vi "Soft_Robot Model.vi"() -> ()   [LabVIEW 2015]
uses:
  <vilib>/addons/Control Design/_Model Construction/Model Typedefs.llb/CD State Space Model (MIMO).ctl
  <vilib>/addons/Control Design/_Model Construction/Model Typedefs.llb/CD General Elements.ctl
  <vilib>/Analysis/Matrix/Datatypes/RealMatrix.ctl
  <vilib>/Platform/TimedLoop/XDataNode/timing_clust.ctl
  <vilib>/Platform/TimedLoop/XDataNode/nitl_modes.ctl
  <vilib>/Platform/TimedLoop/XDataNode/wakeup.ctl
  <vilib>/FPGAPlugInAG/myRIO-1900/niLvFpga_Open_myRIO-1900.vi
  <vilib>/rvi/interface/common/dynamic/niFpgaDynamicAddResources.vi
  <vilib>/Utility/error.llb/Error Cluster From Error Code.vi
  <vilib>/rvi/errors/niLvFpgaAdjustHostInterfaceError.vi
  <vilib>/FPGAPlugInAG/Dynamic/niLvFpga_Close_Dynamic.vi
  <vilib>/addons/Control Design/_Model Construction/Model Creation.llb/Model Creation SubVI/cd_Create State Space Model.vi
  <vilib>/addons/Control Design/_Stochastic Systems/Stochastic Systems.llb/CD Construct Noise Model (Numeric).vi
  <vilib>/Analysis/7linalg.llb/Create Special Real Matrix.vi
  <vilib>/addons/Control Design/_State Feedback Control/State Feedback Control.llb/State Feedback Control SubVis/cd_Linear Quadratic Regulator.vi
  <vilib>/Simulation/Estimation/Implementation/NILVSim Discrete Kalman Filter.llb/SIM Disc KF Pred and Corr with Pred Gain with Checking Direct LV.vi
  <vilib>/rvi/interface/nirviOpenFPGA/nirviOpenFPGA.xnode
  FPGA Bitfiles/ACC20115_FPGATarget_CurrentControlle_Dt5vFgOzYtY.lvbitx
  Current Controller.vi
  <vilib>/rvi/interface/nirviReadWriteControl/nirviReadWriteControl.xnode
  <vilib>/rvi/interface/nirviCloseFPGA/nirviCloseFPGA.xnode
  <vilib>/Platform/TimedLoop/XDataNode/XDataNode.xnode
  <vilib>/Simulation/Implementation/XNodeFramework/SimXNode/SimX.xnode
  NiFpgaLv.dll
  <vilib>/rvi/interface/Simulation/niFpgaSimulationCallBeginRW.vi
  <vilib>/addons/Control Design/_Model Construction/NI_LinSys_Model Creation.lvlib
  <vilib>/addons/Control Design/_State Feedback Control/NI_CD_State Feedback Control.lvlib
  <vilib>/addons/Control Design/_Stochastic Systems/NI_CD_Stochastic Systems.lvlib
  <vilib>/Platform/TimedLoop/XDataNode/XDNodeRunTimeDep.lvlib
  <vilib>/Analysis/NI_AALPro.lvlib
  <vilib>/addons/Control Design/_Model Construction/NI_LinSys_Model Typedefs.lvlib
  <vilib>/Analysis/Matrix/NI_Matrix.lvlib
panel:
  in  "LQR Q":T1
  out "error IO":errorcluster
  in  "Tab Control":enum32{"Outputs/Control", "Model Info"}(tab)
  out "DAC Inlet Valve 2":i32(graph)
  out "Fusion Data":dbl(graph)
  out "KF estimate":dbl[](graph)
  in  "SP1:":dbl(slide)=40.87020302841148 min=0.0 max=0.0 scale=0.0..720.0
  in  "Stop":bool
  in  "LQR Weight (LQR R)":dbl(knob)=1.2163765459278015 scale=1.0..10.0
  out "Status?":bool
  in  "Current (mA)":i32
  out "State-Space Model":T2 {"Transport Delay" format="%.2f"; "D" format="%#.2g"; "C" format="%#.2g"; "B" format="%#.2g"; "A" format="%#.2g"; "properties"."Sampling Time" format="%#.6p"; "properties"."Output Delays" format="%.4f"; "properties"."Input Delays" format="%.4f"}
  in  "A":dbl[][](array[numeric])=[[1.1159, -0.2446, -0.2446, -0.2726], [-0.0103, 0.8088, 0.0684, 0.1117], [-0.167, 0.1085, 0.5344, 0.1174], [0.1346, 0.1551, -0.1383, 0.5146]] format="%#.5g"
  in  "B":dbl[][](array[numeric])=[[-2e-07], [-0.0001119], [-3.4e-06], [0.0001751]] format="%#.5g"
  in  "C":dbl[][](array[numeric])=[[1.494, -0.1725, -0.3513, 0.0724]] format="%#.5g"
  in  "D":dbl[][](array[numeric]) format="%#.5g"
  in  "KF Q":dbl[][](array[numeric])=[[0.01, 0.0], [0.0, 0.001]]
  in  "KF R":dbl[][](array[numeric])=[[0.1]]
  in  "Initial  xhat(0|-1)":dbl[](array[numeric])=[1.0, 0.0]
  in  "Initial  Cov P(0|-1)":dbl[][](array[numeric])=[[1.0, 0.0], [0.0, 1.0]]
  in  "LQR State Weight Matrix (Q)":dbl[](array[slide])=[1.133823501217849, 15.19911082952933] scale=0.001..1000.0
  in  "LQR Output weighting matrix (R)":dbl[](array[slide])=[0.061359072734131735] scale=0.0001..10.0
  out "error out":errorcluster
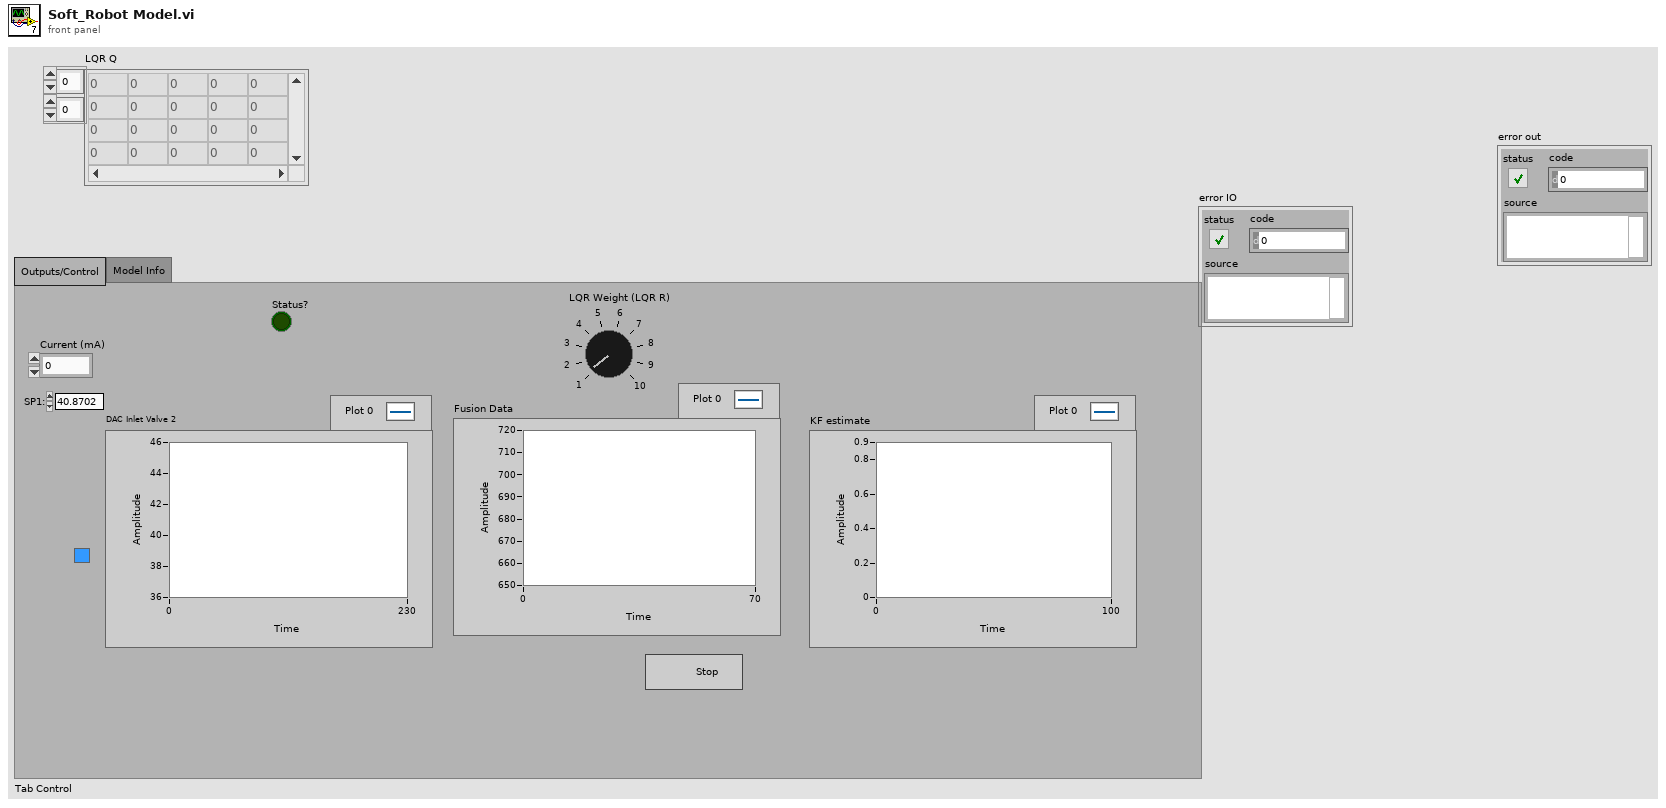
[diagram p1: front panel]
types:
  T1 = typedef "NI_Matrix.lvlib/RealMatrix.ctl" = dbl[][]
  T2 = typedef "NI_LinSys_Model Typedefs.lvlib/CD State Space Model (MIMO).ctl" = cluster{"properties":T3, "A":dbl[][], "B":dbl[][], "C":dbl[][], "D":dbl[][], "StateNames":string[], "Transport Delay":dbl[][]}
  T3 = typedef "NI_LinSys_Model Typedefs.lvlib/CD General Elements.ctl" = cluster{"Model name":string, "Input names":string[], "Output names":string[], "Input Delays":dbl[], "Output Delays":dbl[], "Sampling Time":dbl, "Notes":string}
  T4 = typedef "XDNodeRunTimeDep.lvlib/timing_clust.ctl" = cluster{"Expected End [f-1]":u64, "Actual End [f-1]":u64, "Finished Late? [f-1]":bool, "Expected End [i-1]":u64, "Actual End [i-1]":u64, "Finished Late? [i-1]":bool, "Expected Start [i]":u64, "Actual Start [i]":u64, "Expected Start [f]":u64, "Actual Start [f]":u64, "Source Name":string, "Structure Name":string, "Period":i64, "Deadline":i64, "Offset":i64, "Start":i64, "Priority":i32, "Timeout":i32, "Mode":T5, "Wakeup Reason":T6, "Error":errorcluster, "Source Type":string, "Secondary Source Type":string, "Global End Time":u64, "Global Start Time":u64, "Frame Duration":u64, "Iteration Duration":u64, "Assigned CPU":i32, "I/O Scan Engine Mode":u32}
  T5 = typedef "XDNodeRunTimeDep.lvlib/nitl_modes.ctl" = enum32{"No Change", "Process missed periods, maintain original phase", "Discard missed periods, maintain original phase", "Process missed periods, ignore original phase", "Discard missed periods, ignore original phase"}
  T6 = typedef "XDNodeRunTimeDep.lvlib/wakeup.ctl" = enum32{"Normal", "Aborted", "Asynchronous wakeup", "Timing source error", "Timed loop error", "Timeout"}
  T7 = enum16{"state weighting", "output weighting, Dim Q = Ny", "output weighting, Dim Q = Nx"}
  T8 = enum32{"Identity", "Diagonal", "Toepliz", "Vandermonde", "Companion"}
  T9 = typedef "NI_CD_Stochastic Systems.lvlib/cd_Stochastic State-Space Model.ctl" = cluster{"Sampling Time (s)":dbl, "G":dbl[][], "B":dbl[][], "A":dbl[][], "C":dbl[][], "D":dbl[][], "H":dbl[][]}
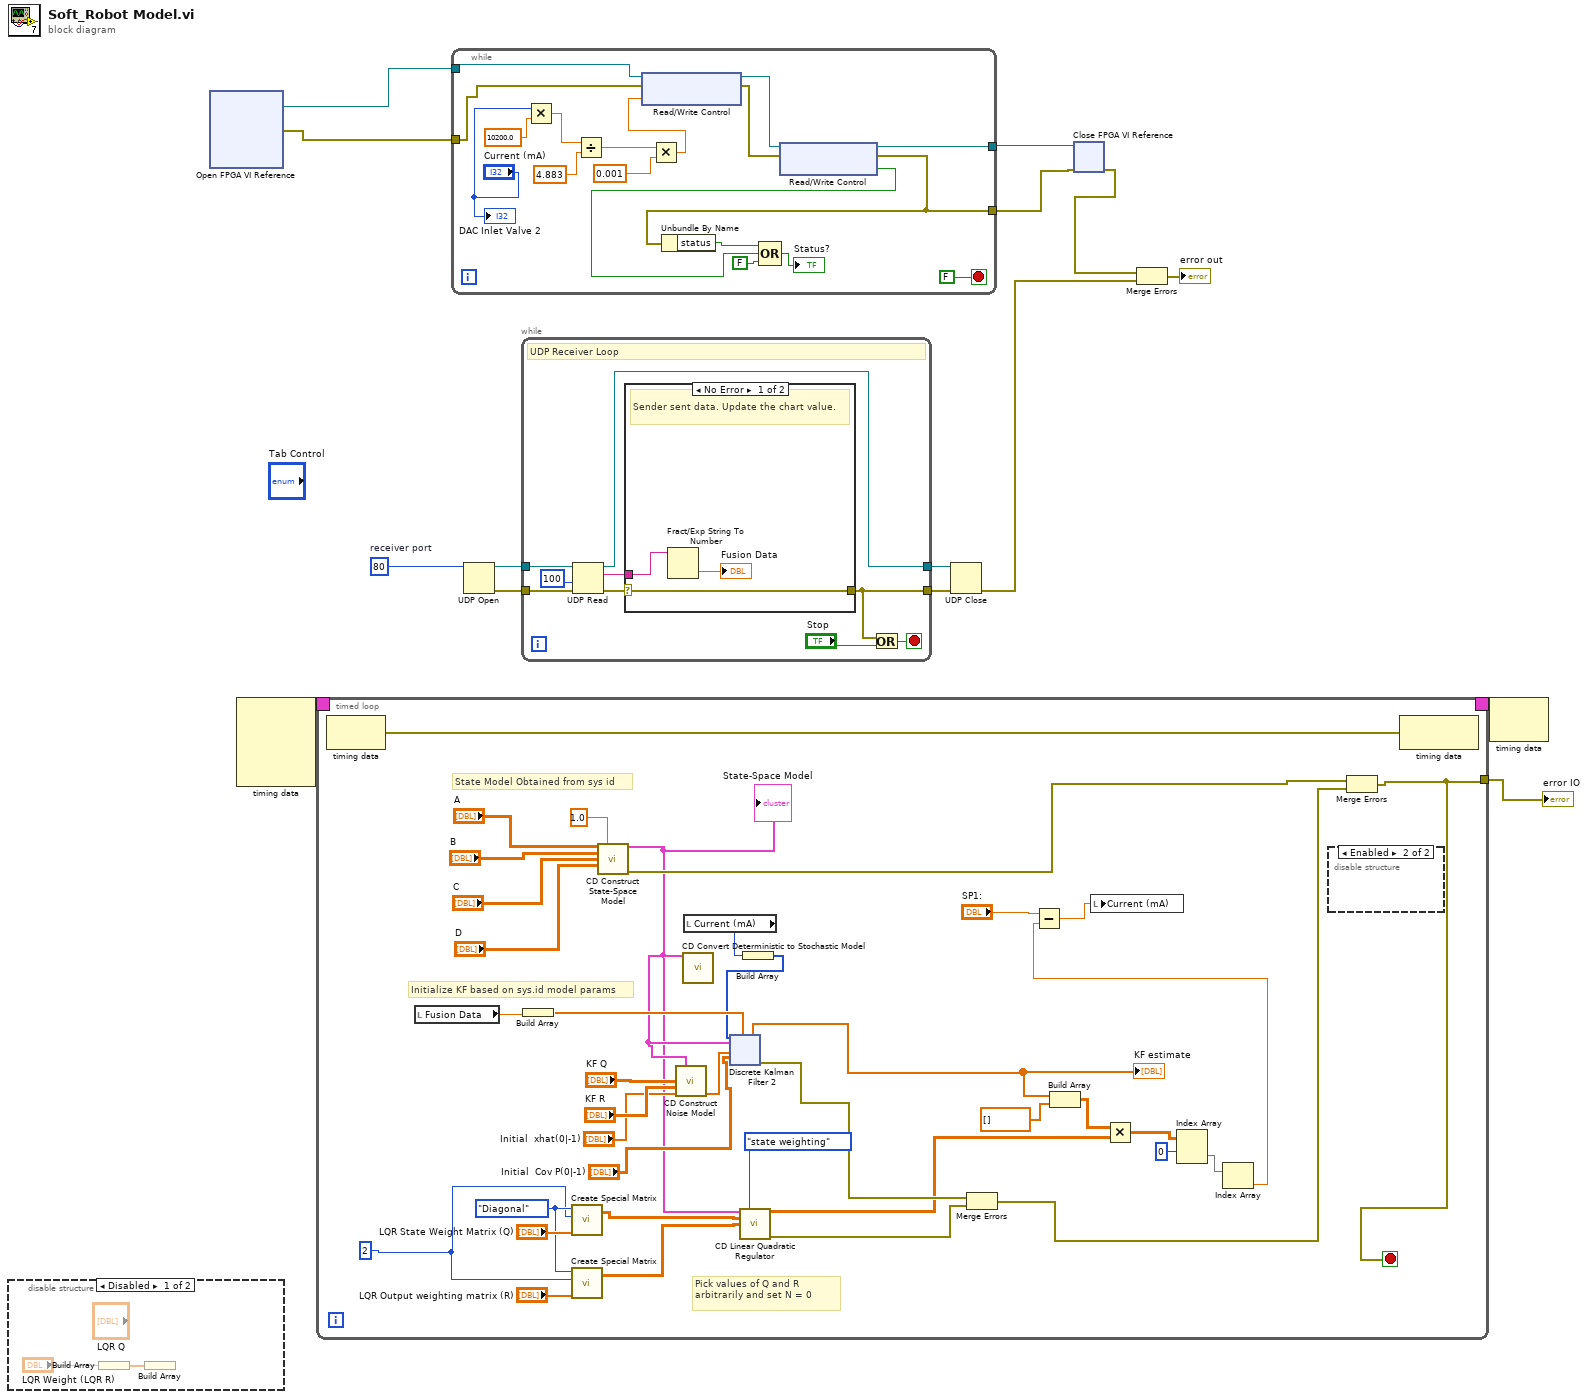
[diagram p0: block diagram]
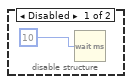
[diagram p3: hidden frame]
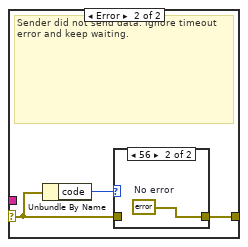
[diagram p4: hidden frame]
diagram:
  w11 = u16 80  # receiver port
  n1 = disable-structure shown="Disabled" {
    frame Disabled {
      n2 = Build Array ("Build Array 3")("LQR Weight (LQR R)") -> (w17:dbl[])
      n3 = Build Array ("Build Array 4")(w17) -> (w18:dbl[][])
    }
    frame Enabled {
    }
  }
  n4 = xnode "Open FPGA VI Reference"() -> ("FPGA VI Reference Out"=w3:refnum<k20>, "error out"=w4:errorcluster)  [unwired: 2 in]
  n5 = node-c288() -> (w2:T4)  [unwired: 4 in]
  n6 = timed-loop {
    tunnel: [w21] -> w5
    timing: w2 -> [_]
    timing-out: [_] -> w1
    stop <- w21 stop-if-true
    w22 = 2
    w29 = T8."Diagonal" ("matrix type")
    # "Pick values of Q and R\narbitrarily and set N = 0"
    # "State Model Obtained from sys id"
    # "Initialize KF based on sys.id model params"
    n7 = node-c288() -> (w20:errorcluster)  [unwired: 1 in]
    n8 = local read "Fusion Data"() -> (w44:dbl)
    n9 = Build Array ("Build Array 6")(w44) -> (w40:dbl[])
    n10 = call-poly <vilib>:"Create Special Matrix.vi"("matrix type"=w29, "matrix size"=w22, "Input Vector1"="LQR State Weight Matrix (Q)") -> ("Special Matrix"=w26:T1)  [unwired: 2 in, 1 out]
    n11 = call-poly <vilib>:"Create Special Matrix.vi"("matrix type"=w29, "matrix size"=w22, "Input Vector1"="LQR Output weighting matrix (R)") -> ("Special Matrix"=w25:T1)  [unwired: 2 in, 1 out]
    n12 = call-poly <vilib>:"CD Construct State-Space Model.vi"("A"="A", "Sampling Time (s)"=1.0, "B"="B", "C"="C", "D"="D") -> ("State-Space Model"=w27:T2, "error out"=w41:errorcluster)  [unwired: 9 in]
    "State-Space Model" <- w27
    n13 = call <vilib>:"CD Convert Deterministic to Stochastic Model.vi"("Deterministic State-Space Model"=w27) -> ("Stochastic State-Space Model"=w36:T9)  [unwired: 13 in, 1 out]
    n14 = call-poly <vilib>:"CD Construct Noise Model.vi"("Stochastic State-Space Model"=w36, "Q"="KF Q", "R"="KF R") -> ()  [unwired: 11 in, 2 out]
    n15 = local read "Current (mA)"() -> (w42:i32)
    n16 = call-poly <vilib>:"CD Linear Quadratic Regulator.vi"("State-Space Model"=w27, "Weighting Type"=T7."state weighting", "Q"=w26, "R"=w25) -> ("Optimal Gain (K)"=w24:dbl[][], "error out"=w23:errorcluster)  [unwired: 8 in, 2 out]
    n17 = Build Array ("Build Array 5")(w42) -> (w32:i32[])
    n18 = xnode ("Discrete Kalman Filter 2")("input u(k)"=w32, "Stochastic State-Space Model"=w36, "Initial State Estimate xhat(0|-1)"="Initial  xhat(0|-1)", "Initial Estimation Error Covariance P(0|-1)"="Initial  Cov P(0|-1)", "Output y(k)"=w40) -> ("Estimated Output yhat(k)"=w39:dbl[], "error out"=w38:errorcluster)  [unwired: 3 in, 6 out]
    "KF estimate" <- w39
    n19 = Merge Errors(w38, w23) -> (w47:errorcluster)
    n20 = Build Array ("Build Array 9")(w39, dbl[] [] ("element")) -> (w53:dbl[][])
    n21 = Multiply(x=w53, y=w24) -> (x*y=w55:dbl[][])
    n22 = Index Array(array=w55, index (row)=0) -> (element=w57:dbl[])  [unwired: 1 in]
    n23 = Index Array ("Index Array 2")(array=w57) -> (element=w45:dbl)  [unwired: 1 in]
    n24 = Subtract(x="SP1:", y=w45) -> (x-y=w43:dbl)
    n25 = local write "Current (mA)"(w43) -> ()
    n26 = disable-structure shown="Enabled" {
      frame Disabled {
        n27 = Wait (ms)(milliseconds to wait=u32 10 ("millisecond timer value")) -> ()  [unwired: 1 out]
      }
      frame Enabled {
      }
    }
    n28 = Merge Errors(w41, w47) -> (w21:errorcluster)
    n29 = node-c288(w20) -> ()  [unwired: 1 out]
  }
  "error IO" <- w5
  n30 = while {
    tunnel: w3 -> [w96]
    tunnel: w4 -> [w80]
    tunnel: [w90] -> w9
    tunnel: [w88] -> w10
    stop <- FALSE stop-if-true
    n31 = Multiply(x="Current (mA)", y=10200.0) -> (x*y=w83:dbl)
    n32 = Divide(x=w83, y=4.883) -> (x/y=w86:dbl)
    n33 = Multiply(x=w86, y=0.001) -> (x*y=w82:dbl)
    n34 = xnode "Read/Write Control"("FPGA VI Reference In"=w96, "error in"=w80, "DAC Inlet Valve"=w82) -> ("FPGA VI Reference Out"=w95:refnum<k20>, "error out"=w94:errorcluster)
    n35 = xnode "Read/Write Control"("FPGA VI Reference In"=w95, "error in"=w94) -> ("FPGA VI Reference Out"=w88:refnum<k20>, "error out"=w90:errorcluster, "Inlet Overflow?"=w89:bool)
    n36 = Unbundle By Name(w90) -> ("status"=w92:bool)
    n37 = Compound Arithmetic op=OR(w92, w89, FALSE ("value")) -> (→"Status?":bool)
    "DAC Inlet Valve 2" <- "Current (mA)"
  }
  n38 = UDP Open(11:w11) -> (port=w12:refnum<k16>, 0:w13:errorcluster)  [unwired: 4 in, 1 out]
  n39 = while {
    tunnel: w12 -> [w106]
    tunnel: [w98] -> w15
    tunnel: w13 -> [w103]
    tunnel: [w99] -> w14
    stop <- w104 stop-if-true
    # "UDP Receiver Loop"
    n40 = UDP Read(connection ID=w106, timeout ms (25000)=100, 8:w103) -> (data out=w101:string, error out=w100:errorcluster, 3:w98:refnum<k16>)  [unwired: 3 out]
    n41 = case shown="No Error" w100 {
      selector: w100 -> [w107 w111]
      tunnel: w101 -> [w109 _]
      tunnel: [w107 w110] -> w99
      frame No Error {
        # "Sender sent data. Update the chart value."
        n42 = Fract/Exp String To Number(string=w109) -> (number=→"Fusion Data":dbl)  [unwired: 3 in, 1 out]
      }
      frame Error {
        # "Sender did not send data. Ignore timeout error and keep waiting."
        n43 = Unbundle By Name(w111) -> ("code"=w112:i32)
        n44 = case shown="56" w112 {
          tunnel: w111 -> [w113 _]
          tunnel: [w113 w114] -> w110
          frame Default {
          }
          frame 56 {
            w114 = errorcluster {"status"=FALSE, "code"=0, "source"=""}  # No error
          }
        }
      }
    }
    n45 = Or(x=w99, y="Stop") -> (x .or. y?=w104:bool)
  }
  n46 = UDP Close(connection ID=w15, 8:w14) -> (error out=w7:errorcluster)  [unwired: 1 out]
  n47 = xnode "Close FPGA VI Reference"("FPGA VI Reference In"=w10, "error in"=w9) -> ("error out"=w8:errorcluster)
  n48 = Merge Errors(w8, w7) -> (→"error out":errorcluster)
  n49 = node-c288(w1) -> ()  [unwired: 1 out]
